vi "Write Element of T.vi"(8 "error in":errorcluster, 9 "T[i]":sgl, 10 "index":i32, 11 "CRDS Cell Data in":refnum<class "CRDS Cell Data.lvclass">) -> (0 "error out":errorcluster, 3 "CRDS Cell Data out":refnum<class "CRDS Cell Data.lvclass">)   [LabVIEW 2011, in "CRDS Cell Data.lvclass"]
uses:
  CRDS Cell Data.lvclass
  CRDS Cell Data.lvclass/CRDS Cell Data.ctl
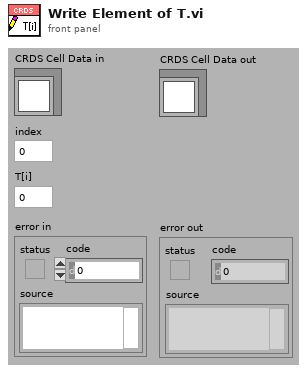
[diagram p1: front panel]
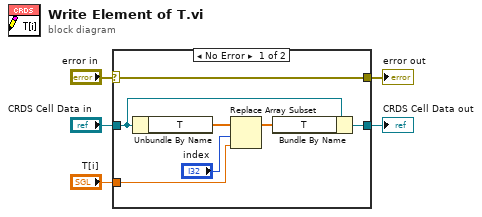
[diagram p0: block diagram]
diagram:
  n1 = case shown="No Error" "error in" {
    selector: "error in" -> [w12 w13]
    tunnel: [w12 w13] -> w4
    tunnel: [w11 w14] -> w2
    tunnel: "CRDS Cell Data in" -> [w10 w14]
    tunnel: "T[i]" -> [w6 _]
    frame No Error {
      n2 = Unbundle By Name(w10) -> ("T"=w9:sgl[])
      n3 = Replace Array Subset(array=w9, new element=w6, index="index") -> (w8:sgl[])
      n4 = Bundle By Name(cluster=w10, "T"=w8) -> (w11:refnum<class "CRDS Cell Data.lvclass">)
    }
    frame Error {
    }
  }
  "error out" <- w4
  "CRDS Cell Data out" <- w2
